vi "getparamcluster.vi"(1 "input cluster":T2) -> (0 "output cluster":T1)   [LabVIEW 2010]
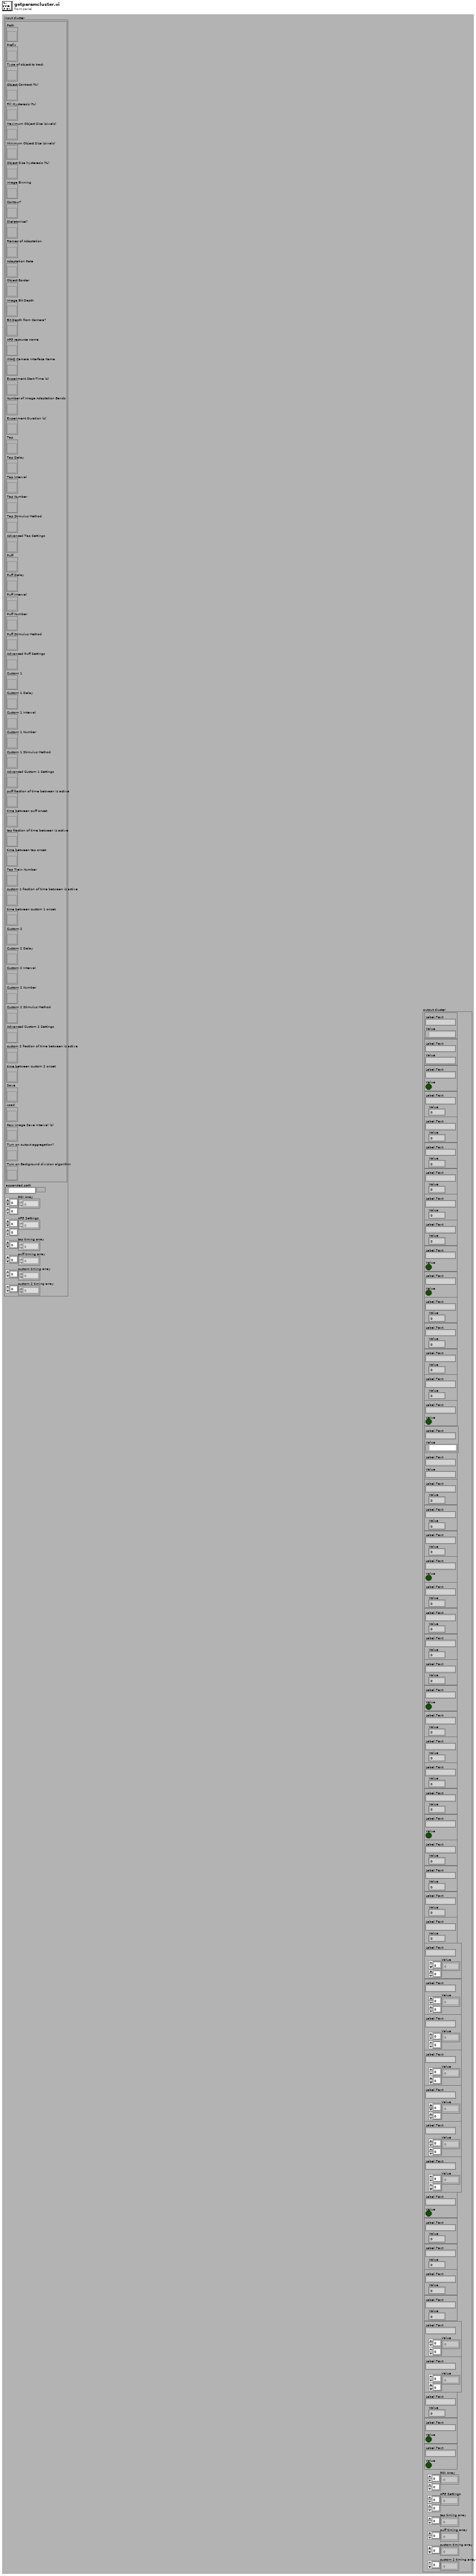
[diagram p1: front panel]
types:
  T1 = cluster{cluster{"Label.Text":string, "Value":path}, cluster{"Label.Text":string, "Value":string}, cluster{"Label.Text":string, "Value":bool}, cluster{"Label.Text":string, "Value":dbl}, cluster{"Label.Text":string, "Value":dbl}, cluster{"Label.Text":string, "Value":i32}, cluster{"Label.Text":string, "Value":i32}, cluster{"Label.Text":string, "Value":dbl}, cluster{"Label.Text":string, "Value":u16}, cluster{"Label.Text":string, "Value":bool}, cluster{"Label.Text":string, "Value":bool}, cluster{"Label.Text":string, "Value":i32}, cluster{"Label.Text":string, "Value":i32}, cluster{"Label.Text":string, "Value":i32}, cluster{"Label.Text":string, "Value":u32}, cluster{"Label.Text":string, "Value":bool}, cluster{"Label.Text":string, "Value":refnum<k15>}, cluster{"Label.Text":string, "Value":string}, cluster{"Label.Text":string, "Value":i32}, cluster{"Label.Text":string, "Value":i32}, cluster{"Label.Text":string, "Value":dbl}, cluster{"Label.Text":string, "Value":bool}, cluster{"Label.Text":string, "Value":dbl}, cluster{"Label.Text":string, "Value":dbl}, cluster{"Label.Text":string, "Value":i32}, cluster{"Label.Text":string, "Value":u16}, cluster{"Label.Text":string, "Value":bool}, cluster{"Label.Text":string, "Value":dbl}, cluster{"Label.Text":string, "Value":dbl}, cluster{"Label.Text":string, "Value":i32}, cluster{"Label.Text":string, "Value":u16}, cluster{"Label.Text":string, "Value":bool}, cluster{"Label.Text":string, "Value":dbl}, cluster{"Label.Text":string, "Value":dbl}, cluster{"Label.Text":string, "Value":i32}, cluster{"Label.Text":string, "Value":u16}, cluster{"Label.Text":string, "Value":sgl[][]}, cluster{"Label.Text":string, "Value":i32[][]}, cluster{"Label.Text":string, "Value":sgl[][]}, cluster{"Label.Text":string, "Value":i32[][]}, cluster{"Label.Text":string, "Value":i32[][]}, cluster{"Label.Text":string, "Value":sgl[][]}, cluster{"Label.Text":string, "Value":i32[][]}, cluster{"Label.Text":string, "Value":bool}, cluster{"Label.Text":string, "Value":dbl}, cluster{"Label.Text":string, "Value":dbl}, cluster{"Label.Text":string, "Value":i32}, cluster{"Label.Text":string, "Value":u16}, cluster{"Label.Text":string, "Value":sgl[][]}, cluster{"Label.Text":string, "Value":i32[][]}, cluster{"Label.Text":string, "Value":dbl}, cluster{"Label.Text":string, "Value":bool}, cluster{"Label.Text":string, "Value":bool}, "ROI Array":dbl[][], "AFG Settings":dbl[][], "tap timing array":dbl[], "puff timing array":dbl[], "custom timing array":dbl[], "custom 2 timing array":dbl[]}
  T2 = cluster{cluster{"Path":refnum<vi>, "Prefix":refnum<vi>, "Type of object to track":refnum<vi>, "Object Contrast (%)":refnum<vi>, "Fill Hysteresis (%)":refnum<vi>, "Maximum Object Size (pixels)":refnum<vi>, "Minimum Object Size (pixels)":refnum<vi>, "Object Size hysteresis (%)":refnum<vi>, "Image Binning":refnum<vi>, "Contour?":refnum<vi>, "Skeletonize?":refnum<vi>, "Frames of Adaptation":refnum<vi>, "Adaptation Rate":refnum<vi>, "Object Border":refnum<vi>, "Image Bit Depth":refnum<vi>, "Bit Depth from Camera?":refnum<vi>, "AFG resource name":refnum<vi>, "IMAQ Camera Interface Name":refnum<vi>, "Experiment Start Time (s)":refnum<vi>, "Number of Image Adaptation Bands":refnum<vi>, "Experiment Duration (s)":refnum<vi>, "Tap":refnum<vi>, "Tap Delay":refnum<vi>, "Tap Interval":refnum<vi>, "Tap Number":refnum<vi>, "Tap Stimulus Method":refnum<vi>, "Advanced Tap Settings":refnum<vi>, "Puff":refnum<vi>, "Puff Delay":refnum<vi>, "Puff Interval":refnum<vi>, "Puff Number":refnum<vi>, "Puff Stimulus Method":refnum<vi>, "Advanced Puff Settings":refnum<vi>, "Custom 1":refnum<vi>, "Custom 1 Delay":refnum<vi>, "Custom 1 Interval":refnum<vi>, "Custom 1 Number":refnum<vi>, "Custom 1 Stimulus Method":refnum<vi>, "Advanced Custom 1 Settings":refnum<vi>, "puff fraction of time between is active":refnum<vi>, "time between puff onset":refnum<vi>, "tap fraction of time between is active":refnum<vi>, "time between tap onset":refnum<vi>, "Tap Train Number":refnum<vi>, "custom 1 fraction of time between is active":refnum<vi>, "time between custom 1 onset":refnum<vi>, "Custom 2":refnum<vi>, "Custom 2 Delay":refnum<vi>, "Custom 2 Interval":refnum<vi>, "Custom 2 Number":refnum<vi>, "Custom 2 Stimulus Method":refnum<vi>, "Advanced Custom 2 Settings":refnum<vi>, "custom 2 fraction of time between is active":refnum<vi>, "time between custom 2 onset":refnum<vi>, "Save":refnum<vi>, "Load":refnum<vi>, "Raw Image Save Interval (s)":refnum<vi>, "Turn on output aggregation?":refnum<vi>, "Turn on Background division algorithm":refnum<vi>}, "appended path":path, "ROI Array":dbl[][], "AFG Settings":dbl[][], "tap timing array":dbl[], "puff timing array":dbl[], "custom timing array":dbl[], "custom 2 timing array":dbl[]}
  T3 = cluster{"Path":refnum<vi>, "Prefix":refnum<vi>, "Type of object to track":refnum<vi>, "Object Contrast (%)":refnum<vi>, "Fill Hysteresis (%)":refnum<vi>, "Maximum Object Size (pixels)":refnum<vi>, "Minimum Object Size (pixels)":refnum<vi>, "Object Size hysteresis (%)":refnum<vi>, "Image Binning":refnum<vi>, "Contour?":refnum<vi>, "Skeletonize?":refnum<vi>, "Frames of Adaptation":refnum<vi>, "Adaptation Rate":refnum<vi>, "Object Border":refnum<vi>, "Image Bit Depth":refnum<vi>, "Bit Depth from Camera?":refnum<vi>, "AFG resource name":refnum<vi>, "IMAQ Camera Interface Name":refnum<vi>, "Experiment Start Time (s)":refnum<vi>, "Number of Image Adaptation Bands":refnum<vi>, "Experiment Duration (s)":refnum<vi>, "Tap":refnum<vi>, "Tap Delay":refnum<vi>, "Tap Interval":refnum<vi>, "Tap Number":refnum<vi>, "Tap Stimulus Method":refnum<vi>, "Advanced Tap Settings":refnum<vi>, "Puff":refnum<vi>, "Puff Delay":refnum<vi>, "Puff Interval":refnum<vi>, "Puff Number":refnum<vi>, "Puff Stimulus Method":refnum<vi>, "Advanced Puff Settings":refnum<vi>, "Custom 1":refnum<vi>, "Custom 1 Delay":refnum<vi>, "Custom 1 Interval":refnum<vi>, "Custom 1 Number":refnum<vi>, "Custom 1 Stimulus Method":refnum<vi>, "Advanced Custom 1 Settings":refnum<vi>, "puff fraction of time between is active":refnum<vi>, "time between puff onset":refnum<vi>, "tap fraction of time between is active":refnum<vi>, "time between tap onset":refnum<vi>, "Tap Train Number":refnum<vi>, "custom 1 fraction of time between is active":refnum<vi>, "time between custom 1 onset":refnum<vi>, "Custom 2":refnum<vi>, "Custom 2 Delay":refnum<vi>, "Custom 2 Interval":refnum<vi>, "Custom 2 Number":refnum<vi>, "Custom 2 Stimulus Method":refnum<vi>, "Advanced Custom 2 Settings":refnum<vi>, "custom 2 fraction of time between is active":refnum<vi>, "time between custom 2 onset":refnum<vi>, "Save":refnum<vi>, "Load":refnum<vi>, "Raw Image Save Interval (s)":refnum<vi>, "Turn on output aggregation?":refnum<vi>, "Turn on Background division algorithm":refnum<vi>}
  T4 = cluster{"Label.Text":string, "Value":refnum<k15>}
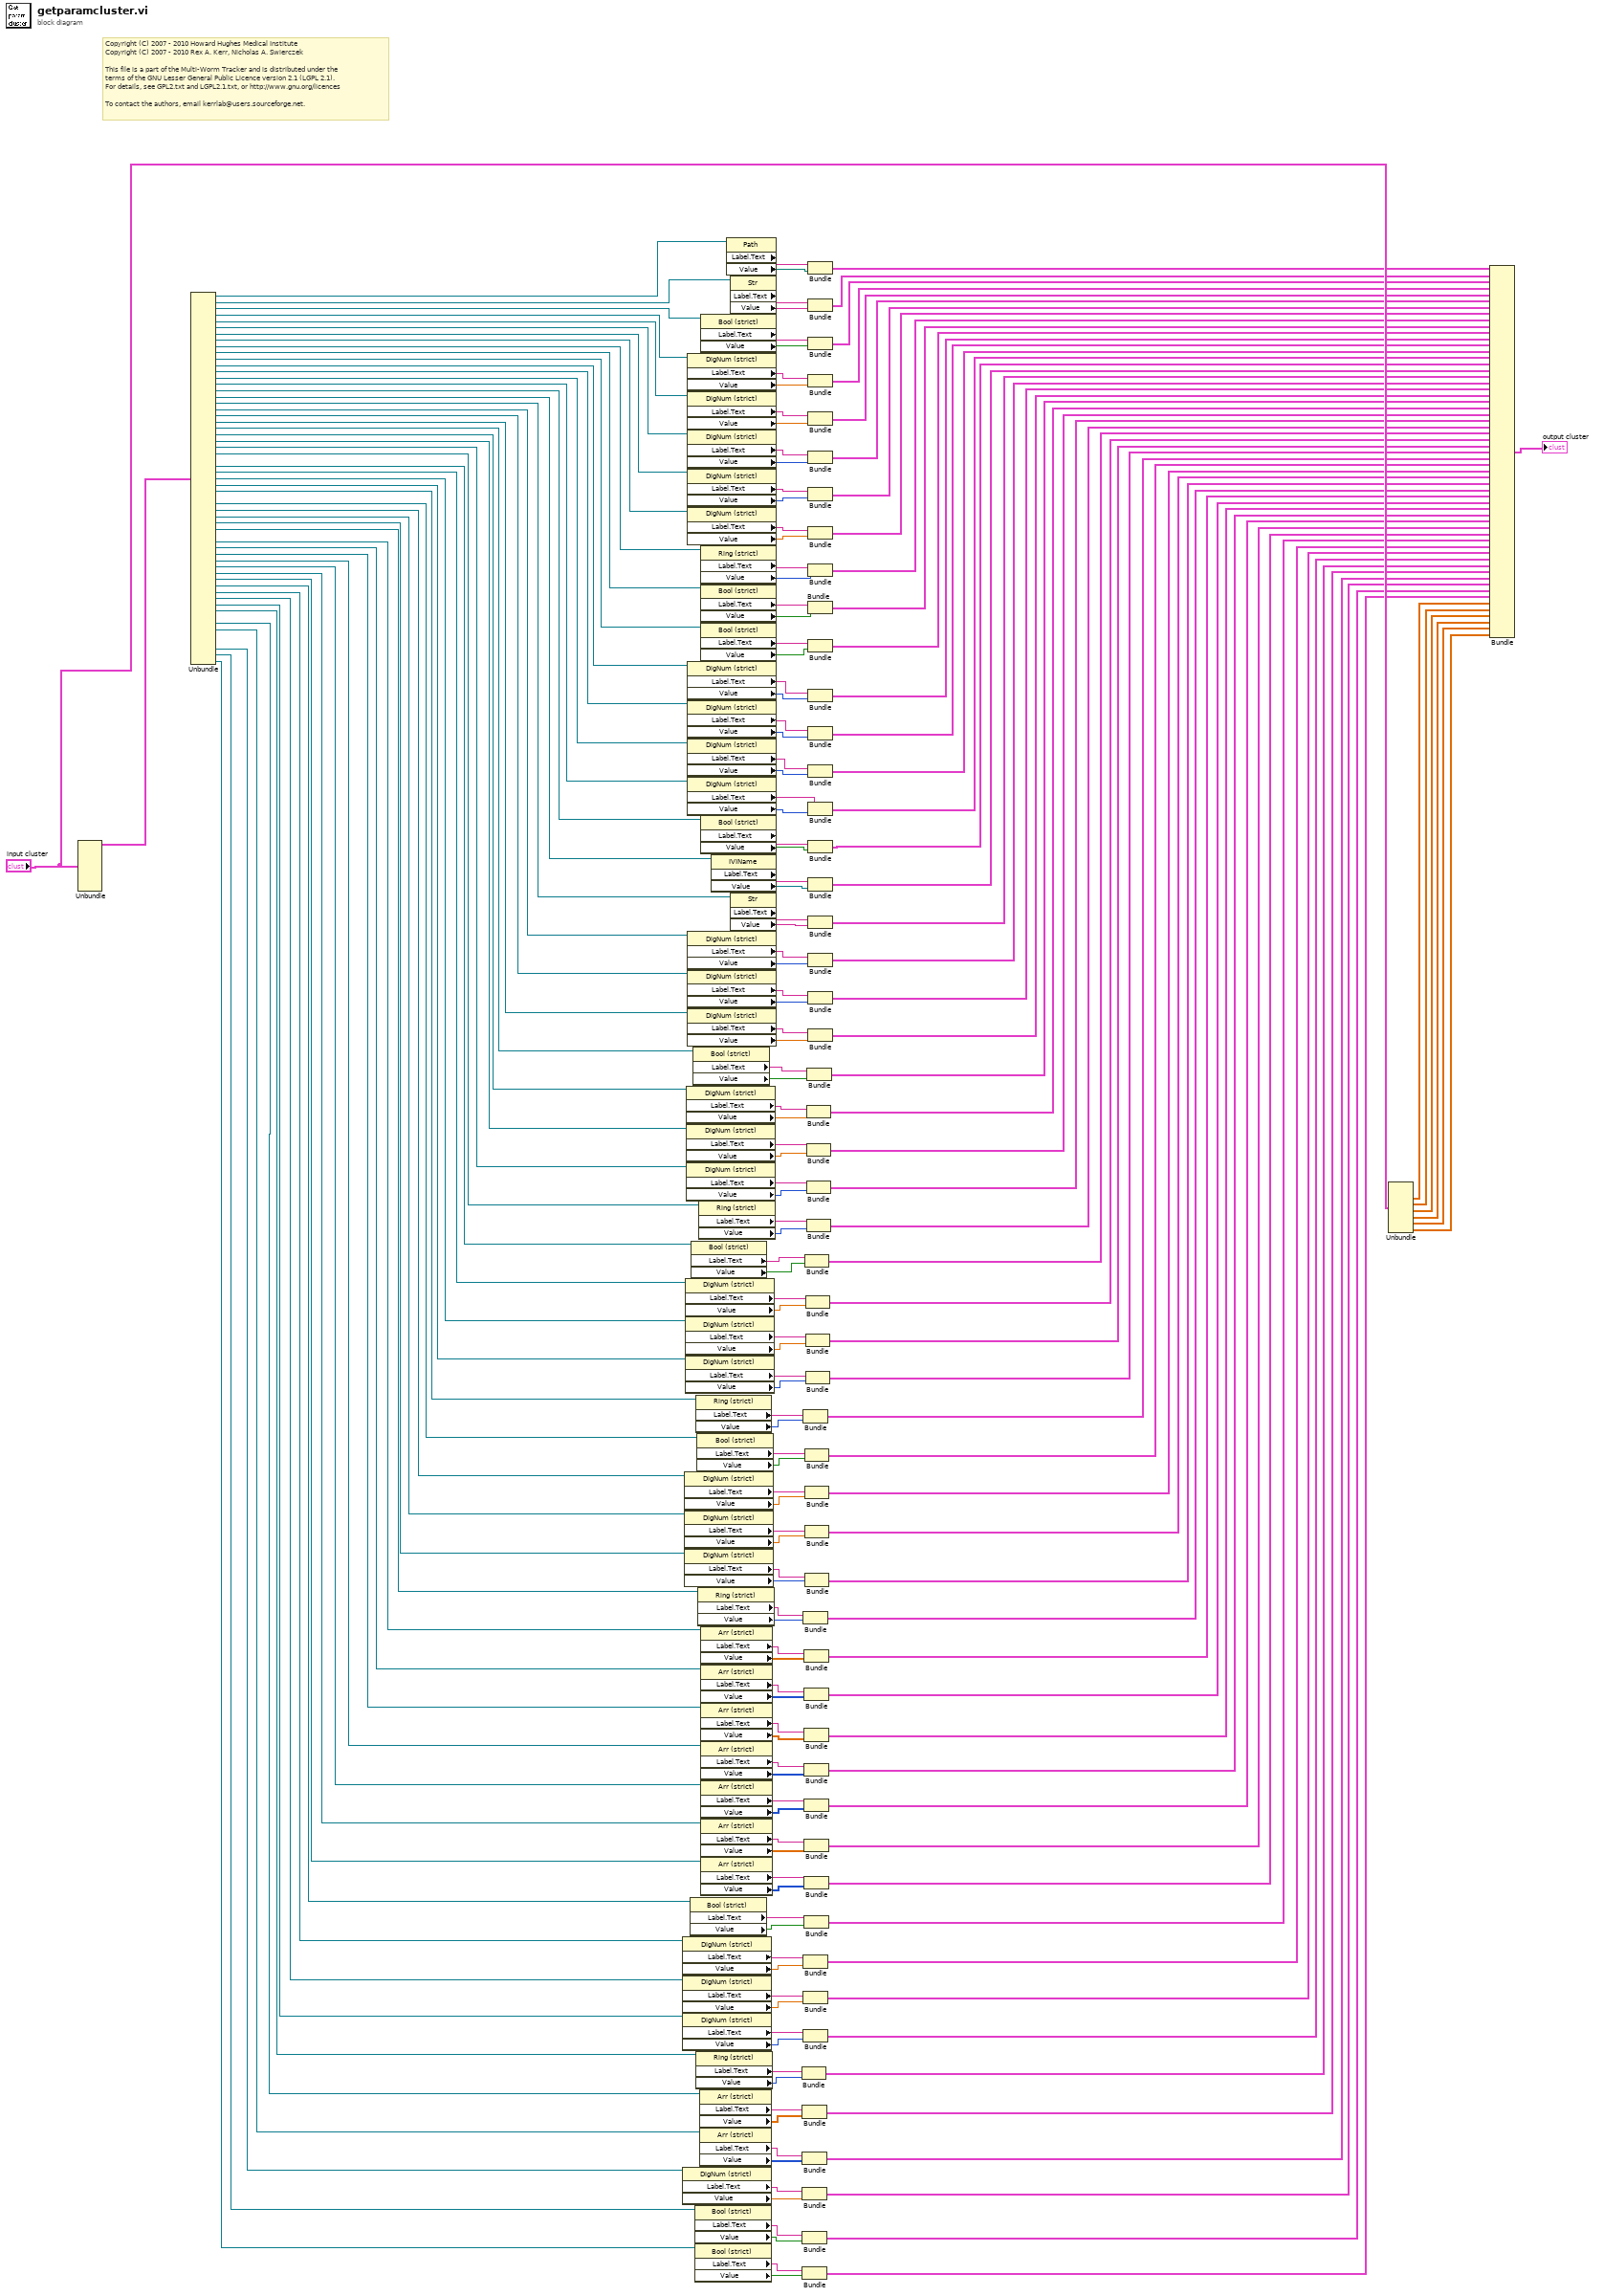
[diagram p0: block diagram]
diagram:
  # "Copyright (C) 2007 - 2010 Howard Hughes Medical Institute\nCopyright (C) 2007 - 2010 Rex A. Kerr, Nicholas A. Swierczek\n \nThis file is a part of the Multi-Worm Tracker and is distributed under the\nterms of the GNU Lesser General Public Licence version 2.1 (LGPL 2.1).\nFor details, see GPL2.txt and LGPL2.1.txt, or http://www.gnu.org/licences\n \nTo contact the authors, email kerrlab@users.sourceforge.net."
  n1 = Unbundle("input cluster") -> (w79:T3)  [unwired: 7 out]
  n2 = Unbundle(w79) -> ("Path"=w221:refnum<vi>, "Prefix"=w220:refnum<vi>, "Type of object to track"=w219:refnum<vi>, "Object Contrast (%)"=w218:refnum<vi>, "Fill Hysteresis (%)"=w217:refnum<vi>, "Maximum Object Size (pixels)"=w216:refnum<vi>, "Minimum Object Size (pixels)"=w215:refnum<vi>, "Object Size hysteresis (%)"=w214:refnum<vi>, "Image Binning"=w213:refnum<vi>, "Contour?"=w212:refnum<vi>, "Skeletonize?"=w211:refnum<vi>, "Frames of Adaptation"=w210:refnum<vi>, "Adaptation Rate"=w209:refnum<vi>, "Object Border"=w208:refnum<vi>, "Image Bit Depth"=w207:refnum<vi>, "Bit Depth from Camera?"=w206:refnum<vi>, "AFG resource name"=w205:refnum<vi>, "IMAQ Camera Interface Name"=w204:refnum<vi>, "Experiment Start Time (s)"=w203:refnum<vi>, "Number of Image Adaptation Bands"=w202:refnum<vi>, "Experiment Duration (s)"=w201:refnum<vi>, "Tap"=w76:refnum<vi>, "Tap Delay"=w200:refnum<vi>, "Tap Interval"=w199:refnum<vi>, "Tap Number"=w198:refnum<vi>, "Tap Stimulus Method"=w197:refnum<vi>, "Puff"=w73:refnum<vi>, "Puff Delay"=w196:refnum<vi>, "Puff Interval"=w195:refnum<vi>, "Puff Number"=w194:refnum<vi>, "Puff Stimulus Method"=w70:refnum<vi>, "Custom 1"=w193:refnum<vi>, "Custom 1 Delay"=w192:refnum<vi>, "Custom 1 Interval"=w191:refnum<vi>, "Custom 1 Number"=w190:refnum<vi>, "Custom 1 Stimulus Method"=w61:refnum<vi>, "puff fraction of time between is active"=w189:refnum<vi>, "time between puff onset"=w188:refnum<vi>, "tap fraction of time between is active"=w187:refnum<vi>, "time between tap onset"=w186:refnum<vi>, "Tap Train Number"=w185:refnum<vi>, "custom 1 fraction of time between is active"=w184:refnum<vi>, "time between custom 1 onset"=w183:refnum<vi>, "Custom 2"=w65:refnum<vi>, "Custom 2 Delay"=w182:refnum<vi>, "Custom 2 Interval"=w181:refnum<vi>, "Custom 2 Number"=w180:refnum<vi>, "Custom 2 Stimulus Method"=w67:refnum<vi>, "custom 2 fraction of time between is active"=w179:refnum<vi>, "time between custom 2 onset"=w178:refnum<vi>, "Raw Image Save Interval (s)"=w177:refnum<vi>, "Turn on output aggregation?"=w176:refnum<vi>, "Turn on Background division algorithm"=w175:refnum<vi>)  [unwired: 6 out]
  n3 = property class="DigNum (strict)"(reference=w177) -> ("Label.Text"=w86:string, "Value"=w85:dbl)  [unwired: 1 in, 2 out]
  n4 = property class="DigNum (strict)"(reference=w182) -> ("Label.Text"=w96:string, "Value"=w95:dbl)  [unwired: 1 in, 2 out]
  n5 = property class="DigNum (strict)"(reference=w181) -> ("Label.Text"=w94:string, "Value"=w93:dbl)  [unwired: 1 in, 2 out]
  n6 = property class="DigNum (strict)"(reference=w180) -> ("Label.Text"=w92:string, "Value"=w91:i32)  [unwired: 1 in, 2 out]
  n7 = property class="DigNum (strict)"(reference=w192) -> ("Label.Text"=w116:string, "Value"=w115:dbl)  [unwired: 1 in, 2 out]
  n8 = property class="DigNum (strict)"(reference=w191) -> ("Label.Text"=w114:string, "Value"=w113:dbl)  [unwired: 1 in, 2 out]
  n9 = property class="DigNum (strict)"(reference=w190) -> ("Label.Text"=w112:string, "Value"=w111:i32)  [unwired: 1 in, 2 out]
  n10 = property class="DigNum (strict)"(reference=w196) -> ("Label.Text"=w124:string, "Value"=w123:dbl)  [unwired: 1 in, 2 out]
  n11 = property class="DigNum (strict)"(reference=w195) -> ("Label.Text"=w122:string, "Value"=w121:dbl)  [unwired: 1 in, 2 out]
  n12 = property class="DigNum (strict)"(reference=w194) -> ("Label.Text"=w120:string, "Value"=w119:i32)  [unwired: 1 in, 2 out]
  n13 = property class="DigNum (strict)"(reference=w200) -> ("Label.Text"=w132:string, "Value"=w131:dbl)  [unwired: 1 in, 2 out]
  n14 = property class="DigNum (strict)"(reference=w199) -> ("Label.Text"=w130:string, "Value"=w129:dbl)  [unwired: 1 in, 2 out]
  n15 = property class="DigNum (strict)"(reference=w198) -> ("Label.Text"=w128:string, "Value"=w127:i32)  [unwired: 1 in, 2 out]
  n16 = property class="DigNum (strict)"(reference=w218) -> ("Label.Text"=w168:string, "Value"=w167:dbl)  [unwired: 1 in, 2 out]
  n17 = property class="DigNum (strict)"(reference=w217) -> ("Label.Text"=w166:string, "Value"=w165:dbl)  [unwired: 1 in, 2 out]
  n18 = property class="DigNum (strict)"(reference=w216) -> ("Label.Text"=w164:string, "Value"=w163:i32)  [unwired: 1 in, 2 out]
  n19 = property class="DigNum (strict)"(reference=w215) -> ("Label.Text"=w162:string, "Value"=w161:i32)  [unwired: 1 in, 2 out]
  n20 = property class="DigNum (strict)"(reference=w214) -> ("Label.Text"=w160:string, "Value"=w159:dbl)  [unwired: 1 in, 2 out]
  n21 = property class="DigNum (strict)"(reference=w210) -> ("Label.Text"=w152:string, "Value"=w151:i32)  [unwired: 1 in, 2 out]
  n22 = property class="DigNum (strict)"(reference=w209) -> ("Label.Text"=w150:string, "Value"=w149:i32)  [unwired: 1 in, 2 out]
  n23 = property class="DigNum (strict)"(reference=w208) -> ("Label.Text"=w148:string, "Value"=w147:i32)  [unwired: 1 in, 2 out]
  n24 = property class="DigNum (strict)"(reference=w207) -> ("Label.Text"=w146:string, "Value"=w145:u32)  [unwired: 1 in, 2 out]
  n25 = property class="DigNum (strict)"(reference=w203) -> ("Label.Text"=w138:string, "Value"=w137:i32)  [unwired: 1 in, 2 out]
  n26 = property class="DigNum (strict)"(reference=w202) -> ("Label.Text"=w136:string, "Value"=w135:i32)  [unwired: 1 in, 2 out]
  n27 = property class="DigNum (strict)"(reference=w201) -> ("Label.Text"=w134:string, "Value"=w133:dbl)  [unwired: 1 in, 2 out]
  n28 = property class="Bool (strict)"(reference=w65) -> ("Label.Text"=w66:string, "Value"=w64:bool)  [unwired: 1 in, 2 out]
  n29 = property class="Bool (strict)"(reference=w73) -> ("Label.Text"=w75:string, "Value"=w74:bool)  [unwired: 1 in, 2 out]
  n30 = property class="Bool (strict)"(reference=w76) -> ("Label.Text"=w78:string, "Value"=w77:bool)  [unwired: 1 in, 2 out]
  n31 = property class="Bool (strict)"(reference=w176) -> ("Label.Text"=w84:string, "Value"=w83:bool)  [unwired: 1 in, 2 out]
  n32 = property class="Bool (strict)"(reference=w175) -> ("Label.Text"=w82:string, "Value"=w81:bool)  [unwired: 1 in, 2 out]
  n33 = property class="Ring (strict)"(reference=w70) -> ("Label.Text"=w71:string, "Value"=w72:u16)  [unwired: 1 in, 2 out]
  n34 = property class="Ring (strict)"(reference=w67) -> ("Label.Text"=w68:string, "Value"=w69:u16)  [unwired: 1 in, 2 out]
  n35 = property class="Bool (strict)"(reference=w193) -> ("Label.Text"=w118:string, "Value"=w117:bool)  [unwired: 1 in, 2 out]
  n36 = property class="Ring (strict)"(reference=w61) -> ("Label.Text"=w62:string, "Value"=w63:u16)  [unwired: 1 in, 2 out]
  n37 = property class="Ring (strict)"(reference=w197) -> ("Label.Text"=w126:string, "Value"=w125:u16)  [unwired: 1 in, 2 out]
  n38 = property class="Arr (strict)"(reference=w179) -> ("Label.Text"=w90:string, "Value"=w89:sgl[][])  [unwired: 1 in, 2 out]
  n39 = property class="Arr (strict)"(reference=w178) -> ("Label.Text"=w88:string, "Value"=w87:i32[][])  [unwired: 1 in, 2 out]
  n40 = property class="Bool (strict)"(reference=w219) -> ("Label.Text"=w170:string, "Value"=w169:bool)  [unwired: 1 in, 2 out]
  n41 = property class="Ring (strict)"(reference=w213) -> ("Label.Text"=w158:string, "Value"=w157:u16)  [unwired: 1 in, 2 out]
  n42 = property class="Bool (strict)"(reference=w212) -> ("Label.Text"=w156:string, "Value"=w155:bool)  [unwired: 1 in, 2 out]
  n43 = property class="Bool (strict)"(reference=w211) -> ("Label.Text"=w154:string, "Value"=w153:bool)  [unwired: 1 in, 2 out]
  n44 = property class="Bool (strict)"(reference=w206) -> ("Label.Text"=w144:string, "Value"=w143:bool)  [unwired: 1 in, 2 out]
  n45 = property class="Arr (strict)"(reference=w189) -> ("Label.Text"=w110:string, "Value"=w109:sgl[][])  [unwired: 1 in, 2 out]
  n46 = property class="Arr (strict)"(reference=w188) -> ("Label.Text"=w108:string, "Value"=w107:i32[][])  [unwired: 1 in, 2 out]
  n47 = property class="Arr (strict)"(reference=w187) -> ("Label.Text"=w106:string, "Value"=w105:sgl[][])  [unwired: 1 in, 2 out]
  n48 = property class="Arr (strict)"(reference=w186) -> ("Label.Text"=w104:string, "Value"=w103:i32[][])  [unwired: 1 in, 2 out]
  n49 = property class="Arr (strict)"(reference=w185) -> ("Label.Text"=w102:string, "Value"=w101:i32[][])  [unwired: 1 in, 2 out]
  n50 = property class="Arr (strict)"(reference=w184) -> ("Label.Text"=w100:string, "Value"=w99:sgl[][])  [unwired: 1 in, 2 out]
  n51 = property class="Arr (strict)"(reference=w183) -> ("Label.Text"=w98:string, "Value"=w97:i32[][])  [unwired: 1 in, 2 out]
  n52 = property class="IVIName"(reference=w205) -> ("Label.Text"=w142:string, "Value"=w141:refnum<k15>)  [unwired: 1 in, 2 out]
  n53 = property class="Path"(reference=w221) -> ("Label.Text"=w174:string, "Value"=w173:path)  [unwired: 1 in, 2 out]
  n54 = property class="Str"(reference=w220) -> ("Label.Text"=w172:string, "Value"=w171:string)  [unwired: 1 in, 2 out]
  n55 = property class="Str"(reference=w204) -> ("Label.Text"=w140:string, "Value"=w139:string)  [unwired: 1 in, 2 out]
  n56 = Bundle("Label.Text"=w68, "Value"=w69) -> (w13:cluster{"Label.Text":string, "Value":u16})  [unwired: 1 in]
  n57 = Bundle("Label.Text"=w90, "Value"=w89) -> (w12:cluster{"Label.Text":string, "Value":sgl[][]})  [unwired: 1 in]
  n58 = Bundle("Label.Text"=w88, "Value"=w87) -> (w11:cluster{"Label.Text":string, "Value":i32[][]})  [unwired: 1 in]
  n59 = Bundle("Label.Text"=w86, "Value"=w85) -> (w10:cluster{"Label.Text":string, "Value":dbl})  [unwired: 1 in]
  n60 = Bundle("Label.Text"=w84, "Value"=w83) -> (w9:cluster{"Label.Text":string, "Value":bool})  [unwired: 1 in]
  n61 = Bundle("Label.Text"=w82, "Value"=w81) -> (w8:cluster{"Label.Text":string, "Value":bool})  [unwired: 1 in]
  n62 = Bundle("Label.Text"=w71, "Value"=w72) -> (w30:cluster{"Label.Text":string, "Value":u16})  [unwired: 1 in]
  n63 = Bundle("Label.Text"=w62, "Value"=w63) -> (w25:cluster{"Label.Text":string, "Value":u16})  [unwired: 1 in]
  n64 = Bundle("Label.Text"=w96, "Value"=w95) -> (w16:cluster{"Label.Text":string, "Value":dbl})  [unwired: 1 in]
  n65 = Bundle("Label.Text"=w94, "Value"=w93) -> (w15:cluster{"Label.Text":string, "Value":dbl})  [unwired: 1 in]
  n66 = Bundle("Label.Text"=w92, "Value"=w91) -> (w14:cluster{"Label.Text":string, "Value":i32})  [unwired: 1 in]
  n67 = Bundle("Label.Text"=w110, "Value"=w109) -> (w24:cluster{"Label.Text":string, "Value":sgl[][]})  [unwired: 1 in]
  n68 = Bundle("Label.Text"=w108, "Value"=w107) -> (w23:cluster{"Label.Text":string, "Value":i32[][]})  [unwired: 1 in]
  n69 = Bundle("Label.Text"=w106, "Value"=w105) -> (w22:cluster{"Label.Text":string, "Value":sgl[][]})  [unwired: 1 in]
  n70 = Bundle("Label.Text"=w104, "Value"=w103) -> (w21:cluster{"Label.Text":string, "Value":i32[][]})  [unwired: 1 in]
  n71 = Bundle("Label.Text"=w102, "Value"=w101) -> (w20:cluster{"Label.Text":string, "Value":i32[][]})  [unwired: 1 in]
  n72 = Bundle("Label.Text"=w100, "Value"=w99) -> (w19:cluster{"Label.Text":string, "Value":sgl[][]})  [unwired: 1 in]
  n73 = Bundle("Label.Text"=w98, "Value"=w97) -> (w18:cluster{"Label.Text":string, "Value":i32[][]})  [unwired: 1 in]
  n74 = Bundle("Label.Text"=w66, "Value"=w64) -> (w17:cluster{"Label.Text":string, "Value":bool})  [unwired: 1 in]
  n75 = Bundle("Label.Text"=w75, "Value"=w74) -> (w34:cluster{"Label.Text":string, "Value":bool})  [unwired: 1 in]
  n76 = Bundle("Label.Text"=w118, "Value"=w117) -> (w29:cluster{"Label.Text":string, "Value":bool})  [unwired: 1 in]
  n77 = Bundle("Label.Text"=w116, "Value"=w115) -> (w28:cluster{"Label.Text":string, "Value":dbl})  [unwired: 1 in]
  n78 = Bundle("Label.Text"=w114, "Value"=w113) -> (w27:cluster{"Label.Text":string, "Value":dbl})  [unwired: 1 in]
  n79 = Bundle("Label.Text"=w112, "Value"=w111) -> (w26:cluster{"Label.Text":string, "Value":i32})  [unwired: 1 in]
  n80 = Bundle("Label.Text"=w124, "Value"=w123) -> (w33:cluster{"Label.Text":string, "Value":dbl})  [unwired: 1 in]
  n81 = Bundle("Label.Text"=w122, "Value"=w121) -> (w32:cluster{"Label.Text":string, "Value":dbl})  [unwired: 1 in]
  n82 = Bundle("Label.Text"=w120, "Value"=w119) -> (w31:cluster{"Label.Text":string, "Value":i32})  [unwired: 1 in]
  n83 = Bundle("Label.Text"=w132, "Value"=w131) -> (w38:cluster{"Label.Text":string, "Value":dbl})  [unwired: 1 in]
  n84 = Bundle("Label.Text"=w130, "Value"=w129) -> (w37:cluster{"Label.Text":string, "Value":dbl})  [unwired: 1 in]
  n85 = Bundle("Label.Text"=w128, "Value"=w127) -> (w36:cluster{"Label.Text":string, "Value":i32})  [unwired: 1 in]
  n86 = Bundle("Label.Text"=w126, "Value"=w125) -> (w35:cluster{"Label.Text":string, "Value":u16})  [unwired: 1 in]
  n87 = Bundle("Label.Text"=w78, "Value"=w77) -> (w39:cluster{"Label.Text":string, "Value":bool})  [unwired: 1 in]
  n88 = Bundle("Label.Text"=w174, "Value"=w173) -> (w60:cluster{"Label.Text":string, "Value":path})  [unwired: 1 in]
  n89 = Bundle("Label.Text"=w172, "Value"=w171) -> (w59:cluster{"Label.Text":string, "Value":string})  [unwired: 1 in]
  n90 = Bundle("Label.Text"=w170, "Value"=w169) -> (w58:cluster{"Label.Text":string, "Value":bool})  [unwired: 1 in]
  n91 = Bundle("Label.Text"=w168, "Value"=w167) -> (w57:cluster{"Label.Text":string, "Value":dbl})  [unwired: 1 in]
  n92 = Bundle("Label.Text"=w166, "Value"=w165) -> (w56:cluster{"Label.Text":string, "Value":dbl})  [unwired: 1 in]
  n93 = Bundle("Label.Text"=w164, "Value"=w163) -> (w55:cluster{"Label.Text":string, "Value":i32})  [unwired: 1 in]
  n94 = Bundle("Label.Text"=w162, "Value"=w161) -> (w54:cluster{"Label.Text":string, "Value":i32})  [unwired: 1 in]
  n95 = Bundle("Label.Text"=w160, "Value"=w159) -> (w53:cluster{"Label.Text":string, "Value":dbl})  [unwired: 1 in]
  n96 = Bundle("Label.Text"=w158, "Value"=w157) -> (w52:cluster{"Label.Text":string, "Value":u16})  [unwired: 1 in]
  n97 = Bundle("Label.Text"=w156, "Value"=w155) -> (w51:cluster{"Label.Text":string, "Value":bool})  [unwired: 1 in]
  n98 = Bundle("Label.Text"=w154, "Value"=w153) -> (w50:cluster{"Label.Text":string, "Value":bool})  [unwired: 1 in]
  n99 = Bundle("Label.Text"=w152, "Value"=w151) -> (w49:cluster{"Label.Text":string, "Value":i32})  [unwired: 1 in]
  n100 = Bundle("Label.Text"=w150, "Value"=w149) -> (w48:cluster{"Label.Text":string, "Value":i32})  [unwired: 1 in]
  n101 = Bundle("Label.Text"=w148, "Value"=w147) -> (w47:cluster{"Label.Text":string, "Value":i32})  [unwired: 1 in]
  n102 = Bundle("Label.Text"=w146, "Value"=w145) -> (w46:cluster{"Label.Text":string, "Value":u32})  [unwired: 1 in]
  n103 = Bundle("Label.Text"=w144, "Value"=w143) -> (w45:cluster{"Label.Text":string, "Value":bool})  [unwired: 1 in]
  n104 = Bundle("Label.Text"=w142, "Value"=w141) -> (w44:T4)  [unwired: 1 in]
  n105 = Bundle("Label.Text"=w140, "Value"=w139) -> (w43:cluster{"Label.Text":string, "Value":string})  [unwired: 1 in]
  n106 = Bundle("Label.Text"=w138, "Value"=w137) -> (w42:cluster{"Label.Text":string, "Value":i32})  [unwired: 1 in]
  n107 = Bundle("Label.Text"=w136, "Value"=w135) -> (w41:cluster{"Label.Text":string, "Value":i32})  [unwired: 1 in]
  n108 = Bundle("Label.Text"=w134, "Value"=w133) -> (w40:cluster{"Label.Text":string, "Value":dbl})  [unwired: 1 in]
  n109 = Unbundle("input cluster") -> ("ROI Array"=w7:dbl[][], "AFG Settings"=w6:dbl[][], "tap timing array"=w5:dbl[], "puff timing array"=w4:dbl[], "custom timing array"=w3:dbl[], "custom 2 timing array"=w2:dbl[])  [unwired: 2 out]
  n110 = Bundle(w60, w59, w58, w57, w56, w55, w54, w53, w52, w51, w50, w49, w48, w47, w46, w45, w44, w43, w42, w41, w40, w39, w38, w37, w36, w35, w34, w33, w32, w31, w30, w29, w28, w27, w26, w25, w24, w23, w22, w21, w20, w19, w18, w17, w16, w15, w14, w13, w12, w11, w10, w9, w8, "ROI Array"=w7, "AFG Settings"=w6, "tap timing array"=w5, "puff timing array"=w4, "custom timing array"=w3, "custom 2 timing array"=w2) -> (→"output cluster":T1)  [unwired: 1 in]
